vi "DSO1072B_FeatchWaveCCW.vi"(11 "VISA resource name In":refnum<visa-resource-name>="USB0::0x0957::0x0588::CN55040452::INSTR") -> (0 "Avg4V8":dbl, 1 "Avg2V9":dbl, 2 "Avg2V1":dbl, 3 "Avg1V3":dbl, 5 "XY Graph CH1":cluster{"Numeric":dbl, "Numeric":dbl}[](graph))   [LabVIEW 2018]
panel:
  out "OutCompare 4":bool
  out "OutCompare 3":bool
  out "OutCompare 2":bool
  out "OutCompare":bool
  out "StartIndeXof2V1":i32
  out "StartIndeXof1V3":i32
  out "StartIndeXof2V9":i32
  out "StartIndeXof4V8":i32
  out "Y-DataCH1":dbl[](array[numeric])
  out "X-DataCH1":dbl[](array[numeric])
  out "yreference":dbl
  out "yorigin":dbl
  out "yincrement":dbl
  out "xreference":dbl
  out "xorigin":dbl
  out "xincrement":dbl format="%#_6f"
  out "NumberOfPoint":i32
  out "<yref>":string
  out "<yorigi>":string
  out "<yinc>":string
  out "<xref>":string
  out "<xorigi>":string
  out "<xinc>":string
  out "<count>":string
  out "<points>":string
  out "<type>":string
  out "<format>":string
  out ":WAV:PRE":string
  out "length":i32
  out "ByteFormatDataCH1":string
  out "data_valueCH1":u8[](array[numeric])
  out "ByteArrayCH1":u8[](array[numeric]) format="%x"
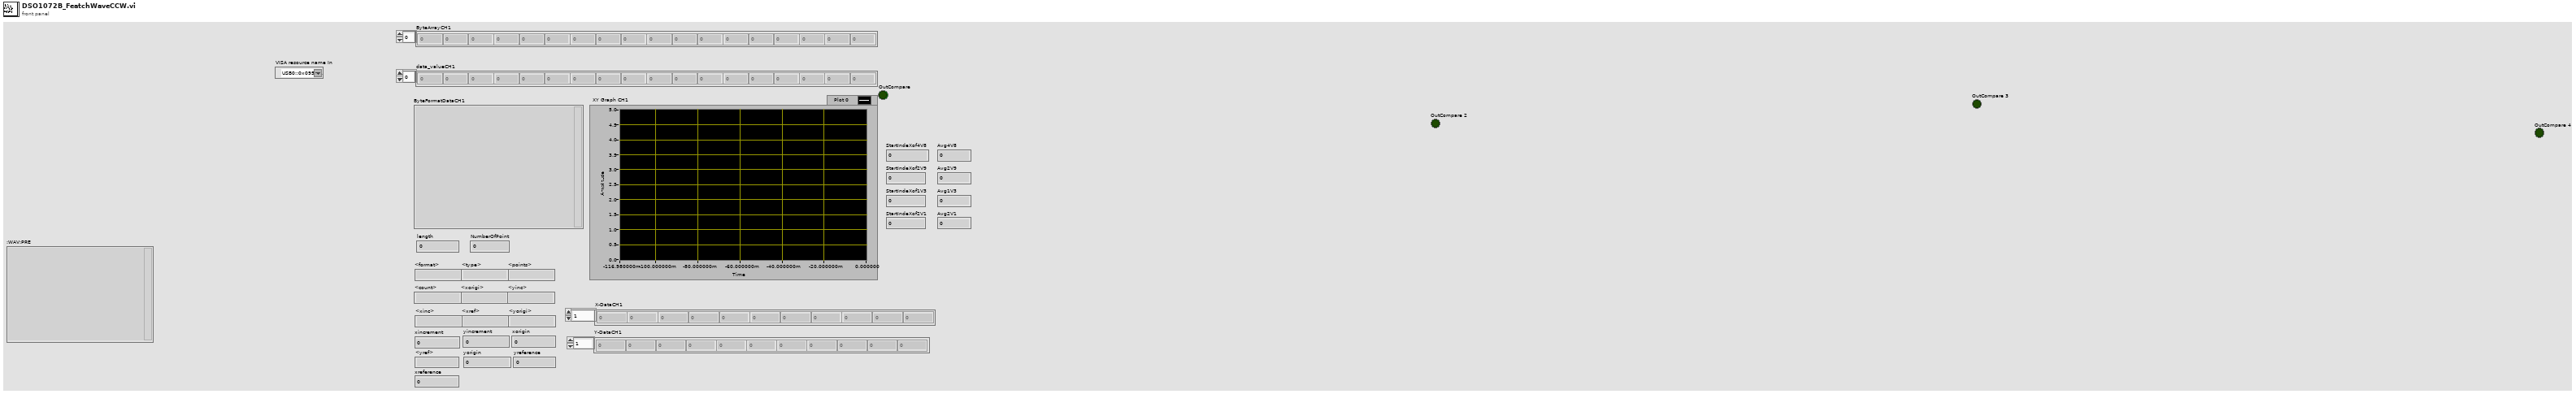
[diagram p1: front panel]
diagram:
  n1 = flat-sequence {
    tunnel: ["VISA resource name In"] -> w13
    tunnel: [w26] -> w14
    tunnel: w13 -> [w26]
    tunnel: [w31] -> w15
    tunnel: w14 -> [w31]
    tunnel: w15 -> [w69]
    tunnel: [w93] -> w12
    tunnel: w12 -> [w111]
    tunnel: [w111] -> w5
    tunnel: [w107] -> w4
    tunnel: [w104] -> w3
    tunnel: w5 -> [w117]
    tunnel: [w117] -> w2
    tunnel: w4 -> [w118]
    tunnel: w3 -> [w116]
    tunnel: w2 -> [w137]
    tunnel: [w137] -> w1
    tunnel: w1 -> [w144]
    tunnel: [w144] -> w11
    tunnel: w11 -> [w161]
    tunnel: [w161] -> w10
    tunnel: w10 -> [w168]
    tunnel: [w168] -> w9
    tunnel: w9 -> [w185]
    tunnel: [w185] -> w8
    tunnel: w8 -> [w192]
    tunnel: [w192] -> w7
    tunnel: w7 -> [w209]
    tunnel: [w209] -> w6
    tunnel: [w221] -> _
    tunnel: w6 -> [w221]
    frame #0 {
      n2 = Initialize Array(0.0 ("element"), 20480 ("dimension size")) -> (→"Y-DataCH1" →"X-DataCH1":dbl[])
    }
    frame #1 {
      n3 = call "DSO1072B_WaveformCMD1.vi"("AutoRead?"=TRUE, "Delay(mS)"=u32 500, "byte count"=u32 20480, "ManualCMD?"=FALSE, "DSO1072B CMD"=":WAV:DATA? CHAN2", "VISA resource name In"="VISA resource name In") -> ("read buffer"=→"ByteFormatDataCH1":string)  [unwired: 3 in, 2 out]
    }
    frame #2 {
      n4 = case shown="True" TRUE {
        frame False {
        }
        frame True {
          n5 = local read "ByteFormatDataCH1"() -> (w29:string)
          n6 = String To Byte Array(string=w29) -> (unsigned byte array=→"ByteArrayCH1":u8[])
          n7 = String Length(string=w29) -> (length=→"length":i32)
        }
      }
    }
    frame #3 {
      w34 = 10 ("index")
      n8 = local read "length"() -> (w35:i32)
      n9 = local read "ByteArrayCH1"() -> (w36:u8[])
      n10 = Subtract(x=w35, y=w34) -> (x-y=w33:i32)
      "NumberOfPoint" <- w33
      n11 = Array Subset(array=w36, index=w34, length=w33) -> (→"data_valueCH1":u8[])
    }
    frame #4 {
      w50 = "," ("regular expression")
      n12 = call "DSO1072B_WaveformCMD1.vi"("AutoRead?"=TRUE, "Delay(mS)"=u32 100, "byte count"=u32 250, "ManualCMD?"=FALSE, "DSO1072B CMD"=":WAV:PRE?", "VISA resource name In"=w69) -> ("read buffer"=w64:string)  [unwired: 3 in, 2 out]
      ":WAV:PRE" <- w64
      n13 = Match Pattern(string=w64, regular expression=w50) -> (before substring=→"<format>":string, after substring=w62:string)  [unwired: 1 in, 2 out]
      n14 = Match Pattern(string=w62, regular expression=w50) -> (before substring=→"<type>":string, after substring=w60:string)  [unwired: 1 in, 2 out]
      n15 = Match Pattern(string=w60, regular expression=w50) -> (before substring=→"<points>":string, after substring=w58:string)  [unwired: 1 in, 2 out]
      n16 = Match Pattern(string=w58, regular expression=w50) -> (before substring=→"<count>":string, after substring=w56:string)  [unwired: 1 in, 2 out]
      n17 = Match Pattern(string=w56, regular expression=w50) -> (before substring=w49:string, after substring=w55:string)  [unwired: 1 in, 2 out]
      "<xinc>" <- w49
      n18 = Match Pattern(string=w55, regular expression=w50) -> (before substring=w47:string, after substring=w54:string)  [unwired: 1 in, 2 out]
      "<xorigi>" <- w47
      n19 = Fract/Exp String To Number(string=w49) -> (number=→"xincrement":dbl)  [unwired: 3 in, 1 out]
      n20 = Match Pattern(string=w54, regular expression=w50) -> (before substring=w44:string, after substring=w53:string)  [unwired: 1 in, 2 out]
      "<xref>" <- w44
      n21 = Fract/Exp String To Number(string=w47) -> (number=→"xorigin":dbl)  [unwired: 3 in, 1 out]
      n22 = Match Pattern(string=w53, regular expression=w50) -> (before substring=w42:string, after substring=w52:string)  [unwired: 1 in, 2 out]
      "<yinc>" <- w42
      n23 = Fract/Exp String To Number(string=w44) -> (number=→"xreference":dbl)  [unwired: 3 in, 1 out]
      n24 = Fract/Exp String To Number(string=w42) -> (number=→"yincrement":dbl)  [unwired: 3 in, 1 out]
      n25 = Match Pattern(string=w52, regular expression=w50) -> (before substring=w40:string, after substring=w51:string)  [unwired: 1 in, 2 out]
      "<yorigi>" <- w40
      n26 = Match Pattern(string=w51, regular expression=w50) -> (before substring=w39:string)  [unwired: 1 in, 3 out]
      "<yref>" <- w39
      n27 = Fract/Exp String To Number(string=w40) -> (number=→"yorigin":dbl)  [unwired: 3 in, 1 out]
      n28 = Fract/Exp String To Number(string=w39) -> (number=→"yreference":dbl)  [unwired: 3 in, 1 out]
    }
    frame #5 {
      # "(YREFerence - data_value)*YINCrement - YORigin"
      # "XORigin + (data_index * XINCrement)"
      n29 = local read "data_valueCH1"() -> (w70:u8[])
      n30 = while {
        tunnel: w70 -> [w92]
        i -> [w74]
        stop <- w76 stop-if-true
        # "(YREFerence – data_value) * YINCrement -YORigin"
        # "XORigin + (data_index * XINCrement)"
        n31 = local read "NumberOfPoint"() -> (w73:i32)
        n32 = local read "yreference"() -> (w85:dbl)
        n33 = local read "yincrement"() -> (w82:dbl)
        n34 = Subtract(x=w73, y=2000) -> (x-y=w71:i32)
        n35 = Index Array(array=w92, index=w74) -> (element=w84:u8)
        n36 = local read "yorigin"() -> (w80:dbl)
        n37 = Equal?(x=w74, y=w71) -> (x = y?=w76:bool)
        n38 = Subtract(x=w85, y=w84) -> (x-y=w83:dbl)
        n39 = local read "xincrement"() -> (w89:dbl)
        n40 = Multiply(x=w83, y=w82) -> (x*y=w81:dbl)
        n41 = Subtract(x=w81, y=w80) -> (x-y=w79:dbl)
        n42 = local read "xorigin"() -> (w91:dbl)
        n43 = Multiply(x=w74, y=w89) -> (x*y=w90:dbl)
        n44 = local read "X-DataCH1"() -> (w88:dbl[])
        n45 = Add(x=w91, y=w90) -> (x+y=w87:dbl)
        n46 = local read "Y-DataCH1"() -> (w86:dbl[])
        n47 = Insert Into Array(array=w88, index=w74, new element=w87) -> (w78:dbl[])
        n48 = Insert Into Array(array=w86, index=w74, new element=w79) -> (w77:dbl[])
        n49 = Build Cluster Array(w78, w77) -> (→"XY Graph CH1":cluster{"Numeric":dbl, "Numeric":dbl}[])
        n50 = local write "X-DataCH1"(w78) -> ()
        n51 = local write "Y-DataCH1"(w77) -> ()
      }
    }
    frame #6 {
      n52 = local read "Y-DataCH1"() -> (w93:dbl[])
      n53 = while {
        tunnel: w93 -> [w102]
        i -> [w97]
        stop <- w96 stop-if-true
        # "Low=4.32\nHigh=5.28"
        # "Find first index of 4V8"
        n54 = Index Array(array=w102, index=w97) -> (element=w101:dbl)
        n55 = local read "NumberOfPoint"() -> (w98:i32)
        n56 = call "CompareMaxMin.vi"("Min"=4.4, "X"=w101, "Max"=5.1) -> ("OutCompare"=w95:bool)
        n57 = case shown="True" w95 {
          tunnel: w97 -> [_ w103]
          frame False {
          }
          frame True {
            "StartIndeXof4V8" <- w103
          }
        }
        n58 = Equal?(x=w97, y=w98) -> (x = y?=w94:bool)
        n59 = Or(x=w95, y=w94) -> (x .or. y?=w96:bool)
      }
    }
    frame #7 {
      w106 = 150 ("length")
      # "101"
      # "100 point to attain stable 4V8 value"
      n60 = local read "StartIndeXof4V8"() -> (w112:i32)
      n61 = Add(x=w112, y=100) -> (x+y=w105:i32)
      n62 = Array Subset(array=w111, index=w105, length=w106) -> (w114:dbl[])
      n63 = Add Array Elements(numeric array=w114) -> (sum=w113:dbl)
      n64 = Add(x=w106, y=w105) -> (x+y=w104:i32)
      n65 = Divide(x=w113, y=w106) -> (x/y=w110:dbl)
      "Avg4V8" <- w110
      n66 = call "CompareMaxMin.vi"("Min"=4.32, "X"=w110, "Max"=5.28) -> ("OutCompare"=w107:bool)
      "OutCompare" <- w107
    }
    frame #8 {
      n67 = case shown="False" w118 {
        tunnel: w117 -> [w120 _]
        tunnel: w116 -> [w119 _]
        frame False {
          n68 = while {
            tunnel: w120 -> [w131]
            tunnel: w119 -> [w122]
            i -> [w123]
            stop <- w126 stop-if-true
            # "Low=4.32\nHigh=5.28"
            # "Find first index of 4V8"
            n69 = Add(x=w123, y=w122) -> (x+y=w121:i32)
            n70 = Index Array(array=w131, index=w121) -> (element=w130:dbl)
            n71 = local read "NumberOfPoint"() -> (w127:i32)
            n72 = call "CompareMaxMin.vi"("Min"=4.4, "X"=w130, "Max"=5.1) -> ("OutCompare"=w125:bool)
            n73 = case shown="True" w125 {
              tunnel: w121 -> [_ w132]
              frame False {
              }
              frame True {
                n74 = local write "StartIndeXof4V8"(w132) -> ()
              }
            }
            n75 = Equal?(x=w121, y=w127) -> (x = y?=w124:bool)
            n76 = Or(x=w125, y=w124) -> (x .or. y?=w126:bool)
          }
        }
        frame True {
        }
      }
    }
    frame #9 {
      w142 = 150 ("length")
      # "101"
      n77 = local read "StartIndeXof4V8"() -> (w141:i32)
      n78 = Add(x=w141, y=100) -> (x+y=w143:i32)
      n79 = Array Subset(array=w137, index=w143, length=w142) -> (w139:dbl[])
      n80 = Add Array Elements(numeric array=w139) -> (sum=w140:dbl)
      n81 = Divide(x=w140, y=w142) -> (x/y=w133:dbl)
      n82 = call "CompareMaxMin.vi"("Min"=4.32, "X"=w133, "Max"=5.28) -> ("OutCompare"=w136:bool)
      n83 = local write "Avg4V8"(w133) -> ()
      n84 = local write "OutCompare"(w136) -> ()
    }
    frame #10 {
      n85 = while {
        tunnel: w144 -> [w155]
        i -> [w151]
        stop <- w147 stop-if-true
        # "Low=1.89\nHigh=2.31"
        # "Find first index of 1V3"
        n86 = local read "StartIndeXof4V8"() -> (w150:i32)
        n87 = Add(x=w151, y=w150) -> (x+y=w145:i32)
        n88 = Index Array(array=w155, index=w145) -> (element=w154:dbl)
        n89 = local read "NumberOfPoint"() -> (w149:i32)
        n90 = call "CompareMaxMin.vi"("Min"=1.9, "X"=w154, "Max"=2.3) -> ("OutCompare"=w146:bool)
        n91 = case shown="True" w146 {
          tunnel: w145 -> [_ w156]
          frame False {
          }
          frame True {
            "StartIndeXof2V1" <- w156
          }
        }
        n92 = Equal?(x=w145, y=w149) -> (x = y?=w148:bool)
        n93 = Or(x=w146, y=w148) -> (x .or. y?=w147:bool)
      }
    }
    frame #11 {
      w166 = 150 ("length")
      # "100 point to attain stable 4V8 value"
      n94 = local read "StartIndeXof2V1"() -> (w167:i32)
      n95 = Add(x=w167, y=100) -> (x+y=w163:i32)
      n96 = Array Subset(array=w161, index=w163, length=w166) -> (w164:dbl[])
      n97 = Add Array Elements(numeric array=w164) -> (sum=w165:dbl)
      n98 = Divide(x=w165, y=w166) -> (x/y=w157:dbl)
      "Avg2V1" <- w157
      n99 = call "CompareMaxMin.vi"("Min"=1.89, "X"=w157, "Max"=2.31) -> ("OutCompare"=→"OutCompare 2":bool)
    }
    frame #12 {
      n100 = while {
        tunnel: w168 -> [w179]
        i -> [w175]
        stop <- w171 stop-if-true
        # "Low=1.17\nHigh=1.43"
        # "Find first index of 1V3"
        n101 = local read "StartIndeXof2V1"() -> (w174:i32)
        n102 = Add(x=w175, y=w174) -> (x+y=w169:i32)
        n103 = Index Array(array=w179, index=w169) -> (element=w178:dbl)
        n104 = local read "NumberOfPoint"() -> (w172:i32)
        n105 = call "CompareMaxMin.vi"("Min"=1.2, "X"=w178, "Max"=1.55) -> ("OutCompare"=w170:bool)
        n106 = case shown="True" w170 {
          tunnel: w169 -> [_ w180]
          frame False {
          }
          frame True {
            "StartIndeXof1V3" <- w180
          }
        }
        n107 = Equal?(x=w169, y=w172) -> (x = y?=w173:bool)
        n108 = Or(x=w170, y=w173) -> (x .or. y?=w171:bool)
      }
    }
    frame #13 {
      w190 = 150 ("length")
      # "100 point to attain stable 4V8 value"
      n109 = local read "StartIndeXof1V3"() -> (w191:i32)
      n110 = Add(x=w191, y=100) -> (x+y=w187:i32)
      n111 = Array Subset(array=w185, index=w187, length=w190) -> (w188:dbl[])
      n112 = Add Array Elements(numeric array=w188) -> (sum=w189:dbl)
      n113 = Divide(x=w189, y=w190) -> (x/y=w181:dbl)
      "Avg1V3" <- w181
      n114 = call "CompareMaxMin.vi"("Min"=1.17, "X"=w181, "Max"=1.43) -> ("OutCompare"=→"OutCompare 3":bool)
    }
    frame #14 {
      n115 = while {
        tunnel: w192 -> [w203]
        i -> [w199]
        stop <- w195 stop-if-true
        # "Low=2.61\nHigh=3.19"
        # "Find first index of 2V9"
        n116 = local read "StartIndeXof1V3"() -> (w198:i32)
        n117 = Add(x=w199, y=w198) -> (x+y=w193:i32)
        n118 = Index Array(array=w203, index=w193) -> (element=w202:dbl)
        n119 = local read "NumberOfPoint"() -> (w196:i32)
        n120 = call "CompareMaxMin.vi"("Min"=2.6, "X"=w202, "Max"=3.1) -> ("OutCompare"=w194:bool)
        n121 = Equal?(x=w193, y=w196) -> (x = y?=w197:bool)
        n122 = case shown="True" w194 {
          tunnel: w193 -> [_ w204]
          frame False {
          }
          frame True {
            "StartIndeXof2V9" <- w204
          }
        }
        n123 = Or(x=w194, y=w197) -> (x .or. y?=w195:bool)
      }
    }
    frame #15 {
      w211 = 150 ("length")
      # "100 point to attain stable 4V8 value"
      n124 = local read "StartIndeXof2V9"() -> (w210:i32)
      n125 = Add(x=w210, y=100) -> (x+y=w214:i32)
      n126 = Array Subset(array=w209, index=w214, length=w211) -> (w213:dbl[])
      n127 = Add Array Elements(numeric array=w213) -> (sum=w212:dbl)
      n128 = Divide(x=w212, y=w211) -> (x/y=w205:dbl)
      "Avg2V9" <- w205
      n129 = call "CompareMaxMin.vi"("Min"=2.61, "X"=w205, "Max"=3.19) -> ("OutCompare"=→"OutCompare 4":bool)
    }
    frame #16 {
      n130 = local read "OutCompare 3"() -> (w218:bool)
      n131 = local read "OutCompare"() -> (w220:bool)
      n132 = local read "OutCompare 4"() -> (w217:bool)
      n133 = local read "OutCompare 2"() -> (w219:bool)
      n134 = Compound Arithmetic op=AND(w220, w219, w218, w217) -> (w216:bool)
      n135 = case shown="False" w216 {
        frame False {
          n136 = Wait (ms)(milliseconds to wait=u32 0) -> ()  [unwired: 1 out]
        }
        frame True {
        }
      }
    }
  }
